vi "earthtilt.vi"(6 "TimeStamp [UT]":timestamp format="%<%H:%M:%S%6u\n%Y/%m/%d>T") -> (0 "dpsi":dbl, 1 "deps":dbl, 2 "eq":dbl, 3 "tobl":dbl, 4 "mobl":dbl)   [LabVIEW 2009]
uses:
  lib/novas-dll.dll
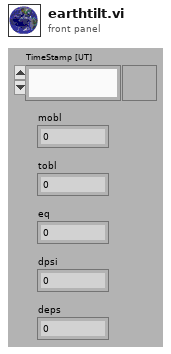
[diagram p1: front panel]
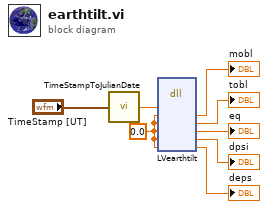
[diagram p0: block diagram]
diagram:
  w8 = 0.0 ("mobl")
  n1 = call "TimeStampToJulianDate.vi"("TimeStamp [UT]"="TimeStamp [UT]") -> ("JulianDay"=w2:ext)
  n2 = dll-call lib="C:/Ohana/LV2009/OhanaOS-LV81/Instruments/Novas/lib/novas-dll.dll" fn="LVearthtilt"("tjd"=w2, "mobl"=w8, "tobl"=w8, "eq"=w8, "dpsi"=w8, "deps"=w8) -> ("mobl"=→"mobl":dbl, "tobl"=→"tobl":dbl, "eq"=→"eq":dbl, "dpsi"=→"dpsi":dbl, "deps"=→"deps":dbl)  [unwired: 3 in, 4 out]
